vi "I2C Read Register (16bit).vi"(8 "error in (no error)":errorcluster, 10 "Register Address":u8, 11 "LINX I2C in":refnum<class "LINX I2C.lvclass">) -> (0 "error out":errorcluster, 2 "Value":u16, 3 "LINX I2C out":refnum<class "LINX I2C.lvclass">)   [LabVIEW 2020, in "LINX I2C.lvclass"]
doc: "Reads a 16-bit register from the I2C device."
uses:
  LINX I2C.lvclass
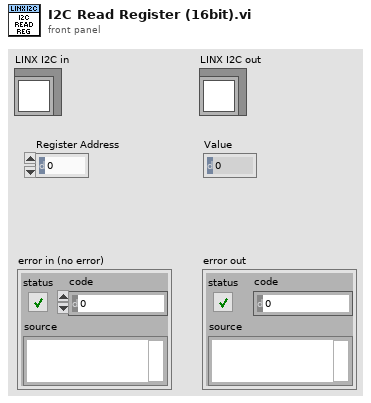
[diagram p1: front panel]
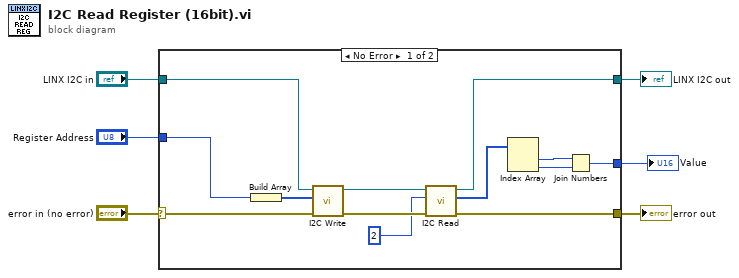
[diagram p0: block diagram]
diagram:
  n1 = case shown="No Error" "error in (no error)" {
    selector: "error in (no error)" -> [w14 w20]
    tunnel: [w12 w21] -> w6
    tunnel: "LINX I2C in" -> [w13 w21]
    tunnel: [w11 w20] -> w4
    tunnel: "Register Address" -> [w15 _]
    tunnel: [w8 _] -> w1
    frame No Error {
      n2 = Build Array(w15) -> (w17:u8[])
      n3 = call "I2C Write.vi"("error in (no error)"=w14, "Bytes to Write"=w17, "LINX I2C in"=w13) -> ("error out"=w19:errorcluster, "LINX I2C out"=w18:refnum<class "LINX I2C.lvclass">)  [unwired: 7 in]
      n4 = call-dynamic "I2C Read.vi"("error in (no error)"=w19, "# Bytes to Read"=u8 2, "LINX I2C in"=w18) -> ("error out"=w11:errorcluster, "Bytes Read"=w7:u8[], "LINX I2C out"=w12:refnum<class "LINX I2C.lvclass">)  [unwired: 6 in]
      n5 = Index Array(array=w7) -> (element #1=w10:u8, element #2=w9:u8)  [unwired: 2 in]
      n6 = Join Numbers(hi=w10, lo=w9) -> ((hi.lo)=w8:u16)
    }
    frame Error {
    }
  }
  "LINX I2C out" <- w6
  "error out" <- w4
  "Value" <- w1
